vi "Generation_singnal.vi"(8 "Phase":dbl, 9 "Amplitude":dbl=1.0, 10 "Frequency":dbl=10.0) -> (3 "Waveform Chart":dynamicdata(graph))   [LabVIEW 2020]
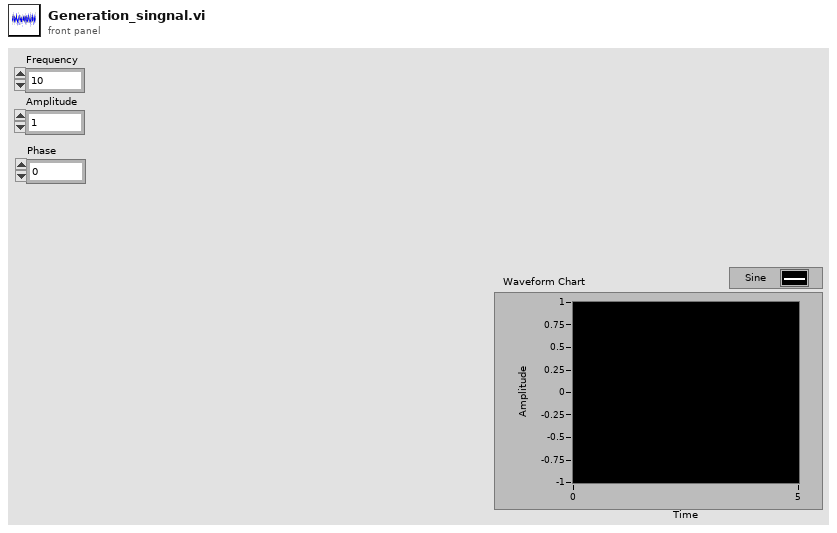
[diagram p1: front panel]
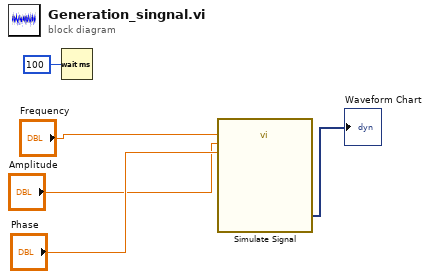
[diagram p0: block diagram]
diagram:
  n1 = Wait (ms)(milliseconds to wait=u32 100) -> ()  [unwired: 1 out]
  n2 = call "Simulate Signal"("Frequency"="Frequency", "Amplitude"="Amplitude", "Phase"="Phase") -> ("Sine"=→"Waveform Chart":dynamicdata)  [unwired: 11 in, 1 out]
